vi "Configure Frequency.vi"(6 "Threshold Voltage Level":dbl min=-700.0 max=700.0, 7 "Aperture Seconds":dbl=0.016667, 8 "error in (no error)":errorcluster, 9 "Threshold Manual Range":dbl=10.0, 10 "Threashold Auto Range? (T: Auto)":bool, 11 "VISA resource name":refnum<visa-resource-name>) -> (0 "error out":errorcluster, 3 "VISA resource name out":refnum<visa-resource-name>)   [LabVIEW 2025, in "Keithley DMM7510.lvlib"]
doc: "This VI configures the Frequency measurement function and related parameters."
uses:
  Keithley DMM7510.lvlib
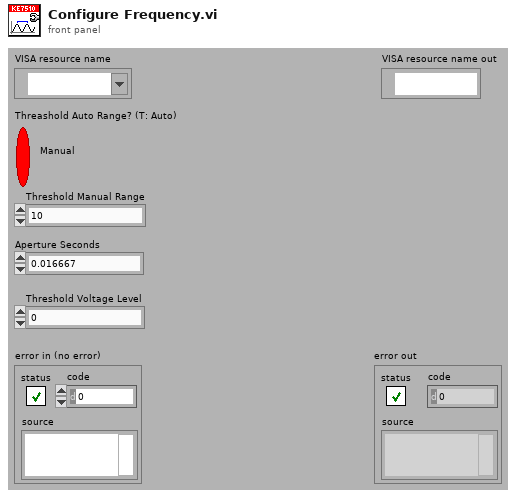
[diagram p1: front panel]
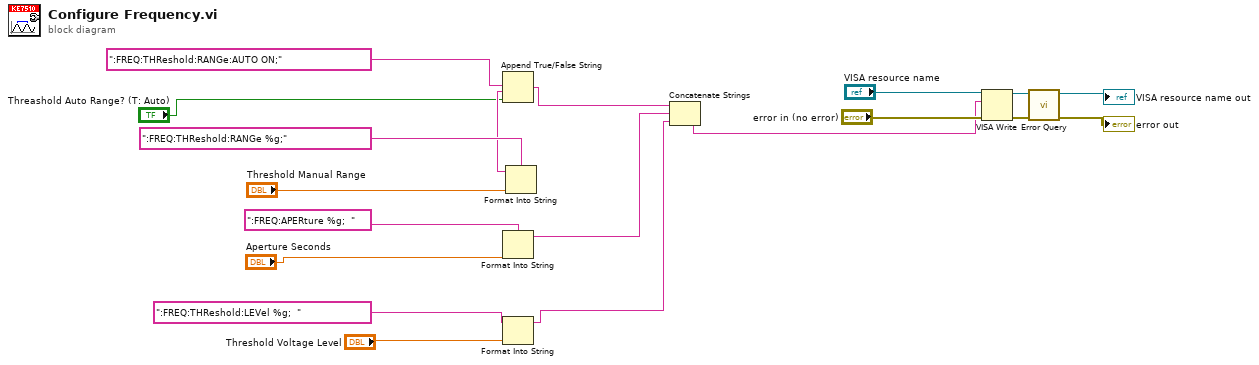
[diagram p0: block diagram]
diagram:
  n1 = Format Into String(format string=":FREQ:APERture %g;  ", "Aperture Seconds") -> (resulting string=w8:string)  [unwired: 2 in, 1 out]
  n2 = Format Into String(format string=":FREQ:THReshold:LEVel %g;  ", "Threshold Voltage Level") -> (resulting string=w1:string)  [unwired: 2 in, 1 out]
  n3 = Format Into String(format string=":FREQ:THReshold:RANGe %g;", "Threshold Manual Range") -> (resulting string=w11:string)  [unwired: 2 in, 1 out]
  n4 = Append True/False String(1:"Threashold Auto Range? (T: Auto)", 2:w11, 3:":FREQ:THReshold:RANGe:AUTO ON;") -> (0:w9:string)  [unwired: 1 in]
  n5 = Concatenate Strings(w9, w8, w1) -> (w7:string)
  n6 = VISA Write(VISA resource name="VISA resource name", write buffer=w7, error in (no error)="error in (no error)") -> (VISA resource name out=w19:refnum<visa-resource-name>, error out=w18:errorcluster)  [unwired: 1 out]
  n7 = call "Error Query.vi"("error in (no error)"=w18, "VISA resource name"=w19) -> ("error out"=→"error out":errorcluster, "VISA resource name out"=→"VISA resource name out":refnum<visa-resource-name>)  [unwired: 6 in, 2 out]
